vi "spawn actor logic.vi"(11 "Template in":refnum<class "Template.lvclass">) -> (0 "error out":errorcluster, 2 "Map":T1(c390), 3 "Template out":refnum<class "Template.lvclass">)   [LabVIEW 2020, in "Template.lvlib" / "Template.lvclass"]
doc: "Creates a map containing all of the nested actors defined in the configuration file and in the ActorConfiguration cluster and generates a map with unique keys for each channel configured through the settings/JSON file"
uses:
  Template.lvclass
  C:/Program Files/National Instruments/LabVIEW 2020/vi.lib/ActorFramework/Actor/Actor.lvclass
  <vilib>/ActorFramework/Message Enqueuer/Message Enqueuer.lvclass
  Template.lvclass/Template.ctl
  <vilib>/regexp/Match Regular Expression.xnode
  <vilib>/ActorFramework/Actor/Actor.lvclass
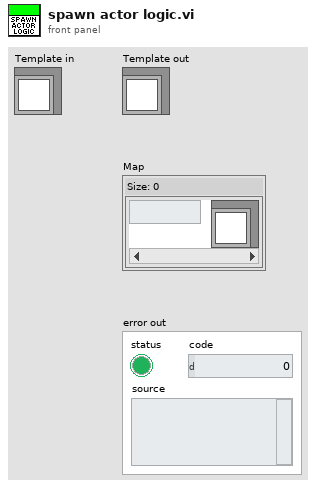
[diagram p1: front panel]
types:
  T1 = map{string, refnum<class "Message Enqueuer.lvclass">}
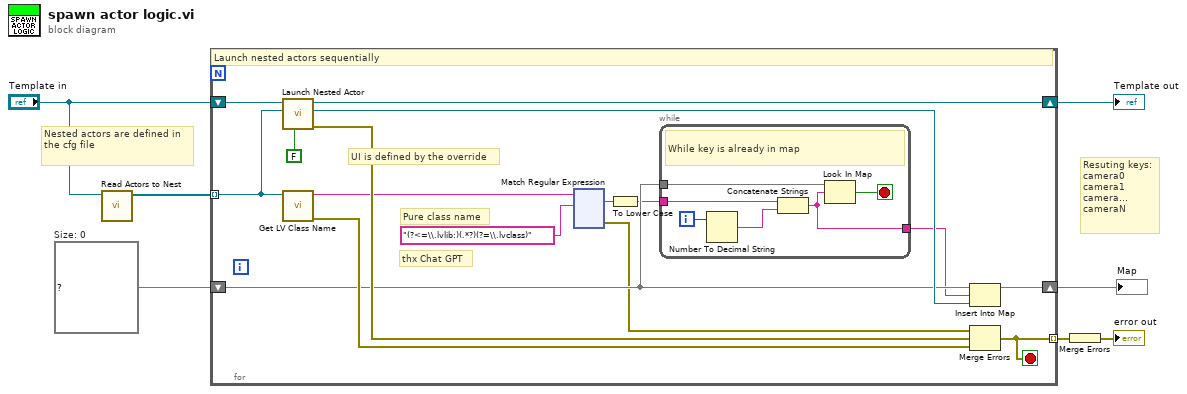
[diagram p0: block diagram]
diagram:
  w6 = T1 {}  # Size: 0
  # "Resuting keys:\ncamera0\ncamera1\ncamera...\ncameraN"
  # "Nested actors are defined in the cfg file"
  n1 = call "Read Actors to Nest.vi"("Template in"="Template in") -> ("Actors to Nest"=w1:refnum<class "Actor.lvclass">[])  [unwired: 10 in]
  n2 = for {
    tunnel: w1 -> [w18] mode=indexing
    shift-right: [w22] -> w4
    shift-left: "Template in" -> [w23]
    shift-right: [w20] -> w5
    shift-left: w6 -> [w15]
    tunnel: [w16] -> w7 mode=indexing
    stop <- w16 stop-if-true
    # "UI is defined by the override"
    # "thx Chat GPT"
    # "Pure class name"
    # "Launch nested actors sequentially"
    n3 = call <vilib>:"Launch Nested Actor.vi"("Open Actor Core front panel? (F)"=FALSE, "Nested Actor"=w18, "Caller Actor in"=w23) -> ("error out"=w19:errorcluster, "Nested Actor's Enqueuer"=w21:refnum<class "Message Enqueuer.lvclass">, "Caller Actor out"=w22:refnum<class "Template.lvclass">)  [unwired: 6 in]
    n4 = call <vilib>:"Get LV Class Name.vi"("object"=w18) -> ("error out"=w17:errorcluster, "class name"=w14:string)  [unwired: 9 in]
    n5 = xnode "Match Regular Expression"("input string"=w14, "regular expression"="(?<=\\.lvlib:)(.*?)(?=\\.lvclass)") -> ("whole match"=w12:string, "error out"=w11:errorcluster)  [unwired: 4 in, 3 out]
    n6 = To Lower Case(string=w12) -> (all lower case string=w10:string)
    n7 = while {
      tunnel: w15 -> [w143]
      tunnel: w10 -> [w142]
      tunnel: [w138] -> w9
      i -> [w140]
      stop <- w141 stop-if-true
      # "While key is already in map"
      n8 = Number To Decimal String(number=w140) -> (decimal integer string=w139:string)  [unwired: 1 in]
      n9 = Concatenate Strings(w142, w139) -> (w138:string)
      n10 = Look In Map(map=w143, key=w138) -> (key not found?=w141:bool)  [unwired: 1 in, 1 out]
    }
    n11 = Insert Into Map(map in=w15, key=w9, value=w21) -> (map out=w20:T1)  [unwired: 2 out]
    n12 = Merge Errors(w11, w19, w17) -> (w16:errorcluster)
  }
  "Template out" <- w4
  "Map" <- w5
  n13 = Merge Errors(w7) -> (→"error out":errorcluster)
